vi "EOL CAN_Init CAL.vi"(7 "Flash Size":i32, 8 "Glass?":bool=TRUE, 9 "Read Session in":refnum<k21>, 10 "DSC Write Session in":refnum<k21>, 11 "SA2 Operator":T1[](array[typedef]) {"Wert" format="%.0x"}) -> (1 "Error String Out":string, 2 "TxRx Data":string[][](array[string]), 3 "Response Good?":bool)   [LabVIEW 2014]
uses:
  Typedefs/Diagnose_SA2_Rechnenbefehl.ctl
  Typedefs/Diagnose_SA2_Operation_ENUM.ctl
  Typedefs/Select Session.ctl
  <vilib>/xnet/xnet.llb/XNET Frame CAN.ctl
  <vilib>/xnet/xnet.llb/XNET Frame Type CAN.ctl
panel:
  in  "Error String":string
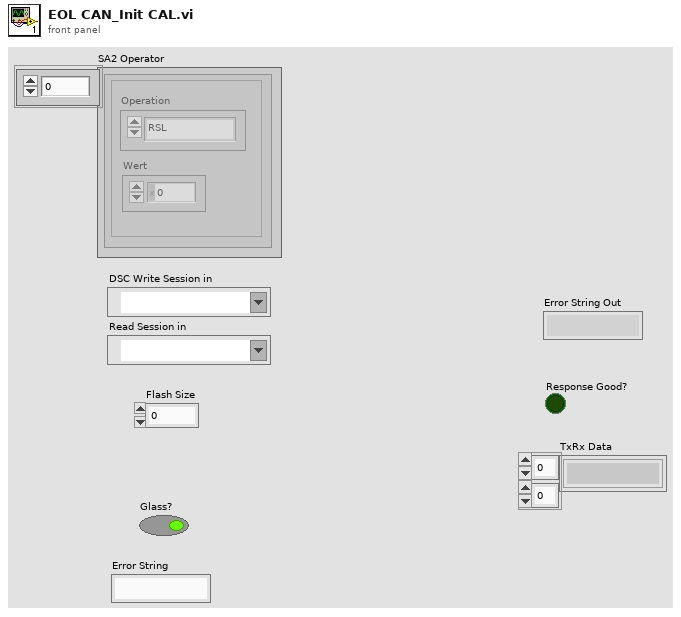
[diagram p1: front panel]
types:
  T1 = typedef "Diagnose_SA2_Rechnenbefehl.ctl" = cluster{"Operation":T2, "Wert":u32}
  T2 = typedef "Diagnose_SA2_Operation_ENUM.ctl" = enum16{"RSL", "RSR", "ADD", "SUB", "EOR", "Durchläufe", "NEXT", "BCC", "BRA", "Fertig"}
  T3 = cluster{"DSC Write Session in":refnum<k21>, "Read Session in":refnum<k21>, "Error String":string, "Response Good?":bool, "Glass?":bool, "TxRx Data":string[][], "SA2 Operator":T1[], "Flash Size":i32}
  T4 = typedef "Select Session.ctl" = enum16{"DefaultSession", "Development", "Extended", "EOL", "Programming"}
  T5 = typedef "XNET Frame CAN.ctl" = cluster{"timestamp":timestamp, "payload":u8[], "identifier":u32, "type":T6, "extended?":bool, "echo?":bool}
  T6 = typedef "XNET Frame Type CAN.ctl" = u8
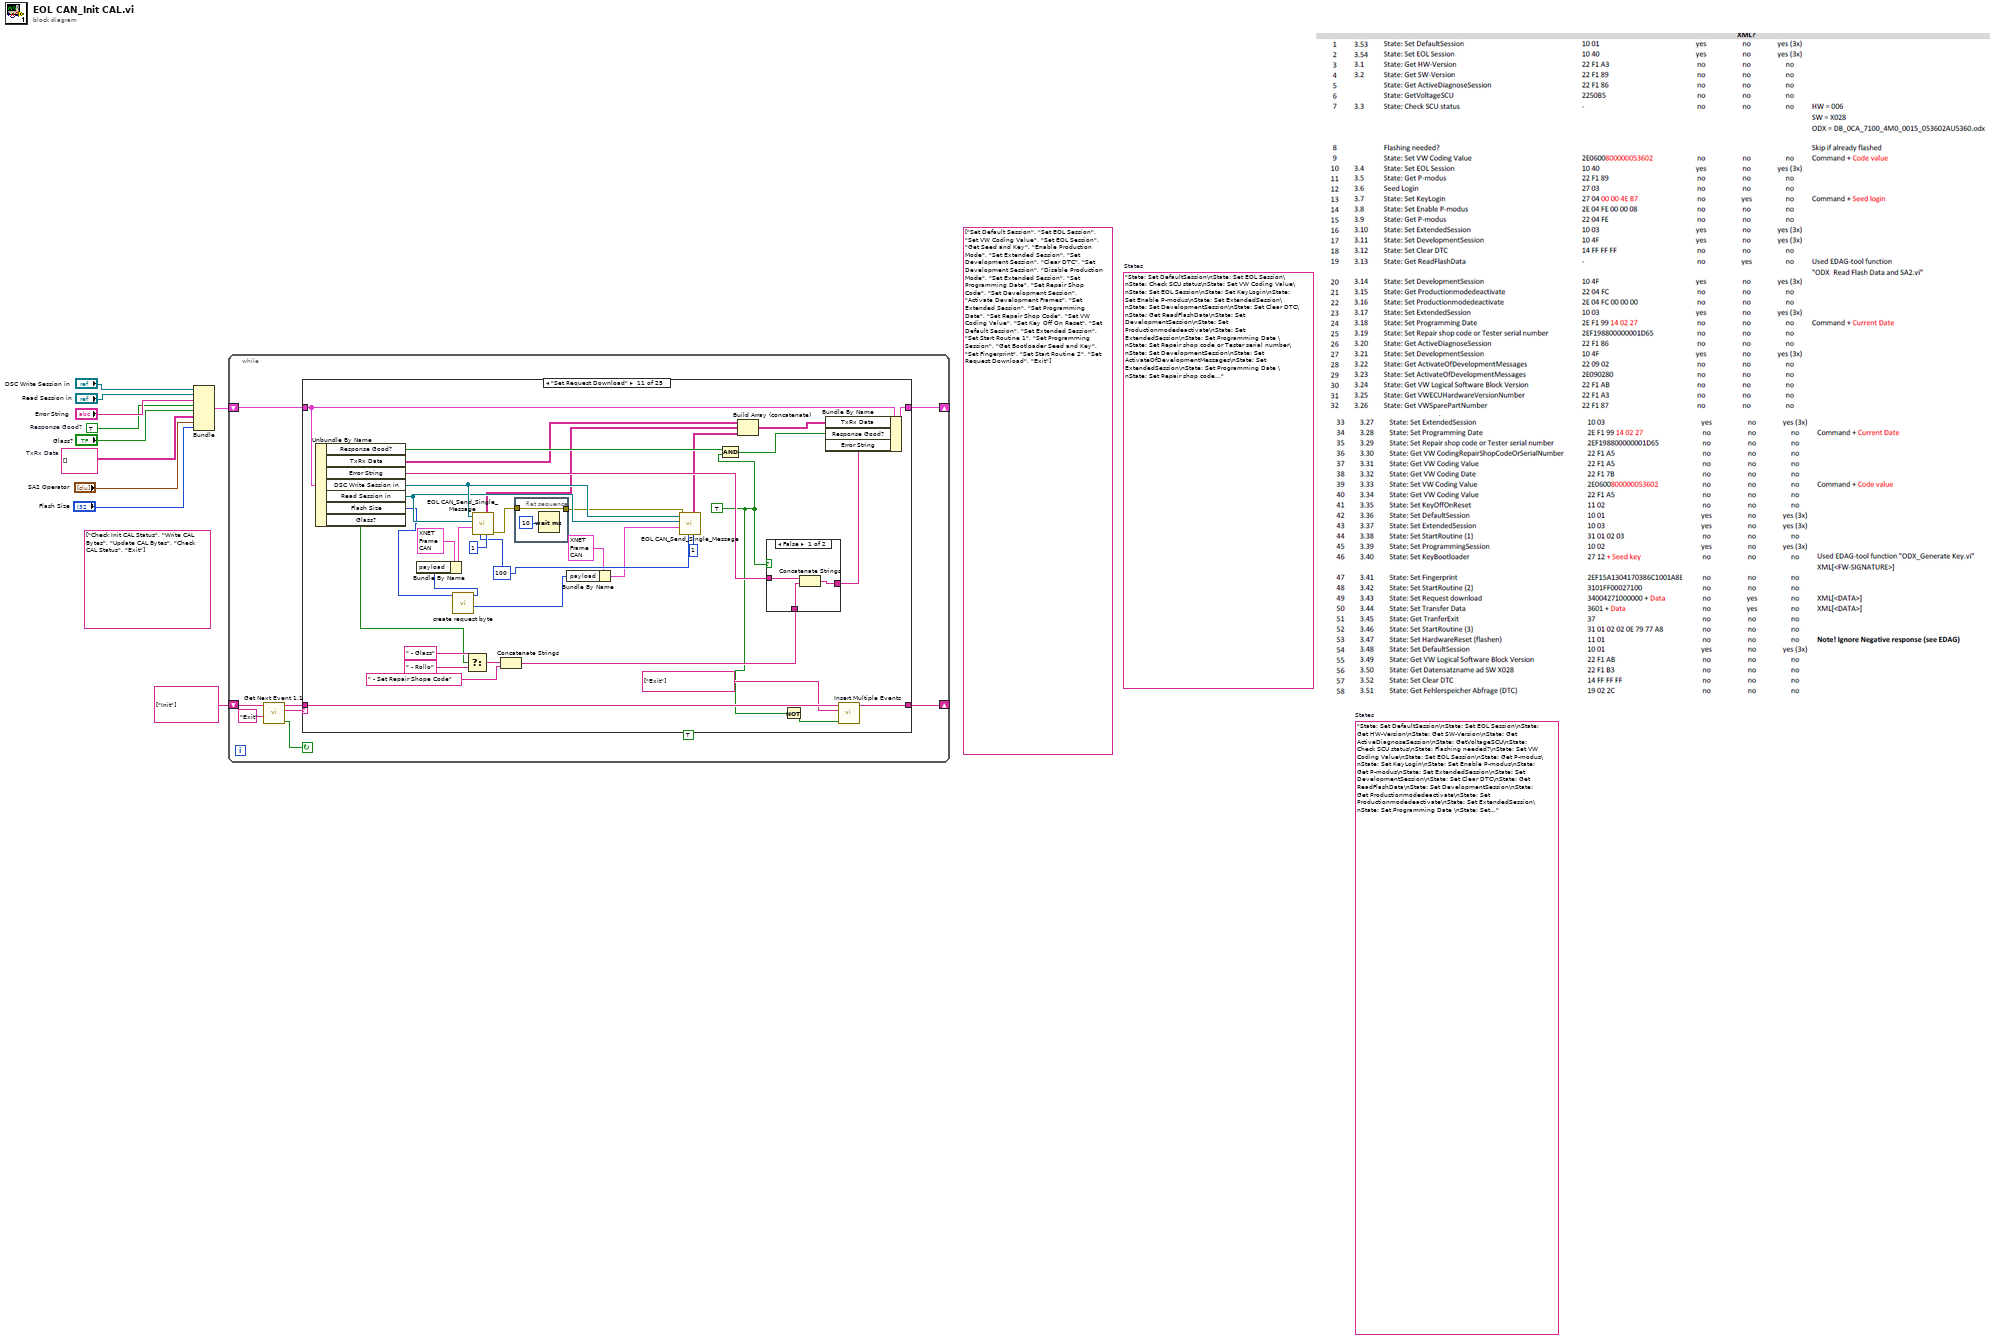
[diagram p0: block diagram]
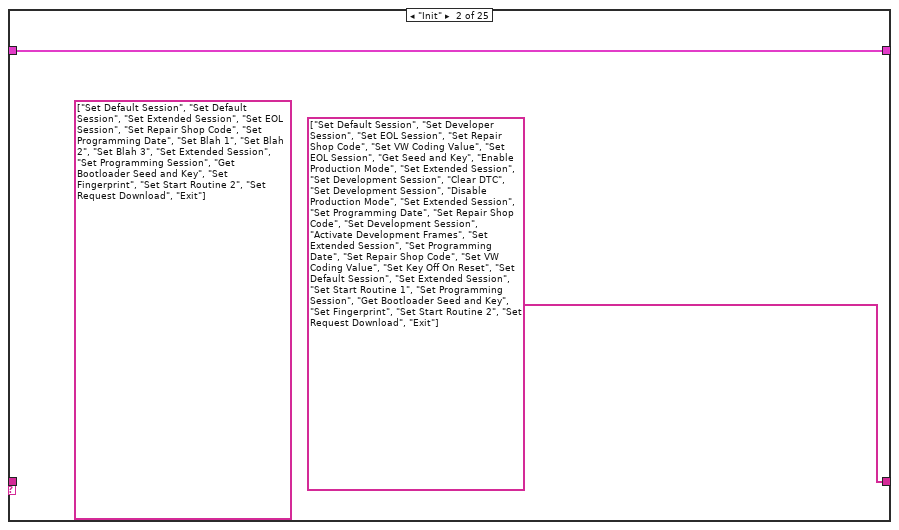
[diagram p3: hidden frame]
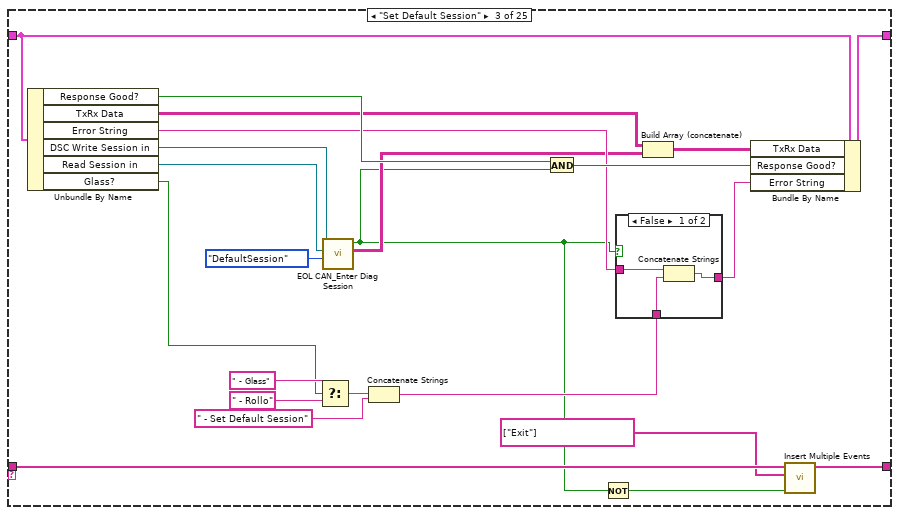
[diagram p4: hidden frame]
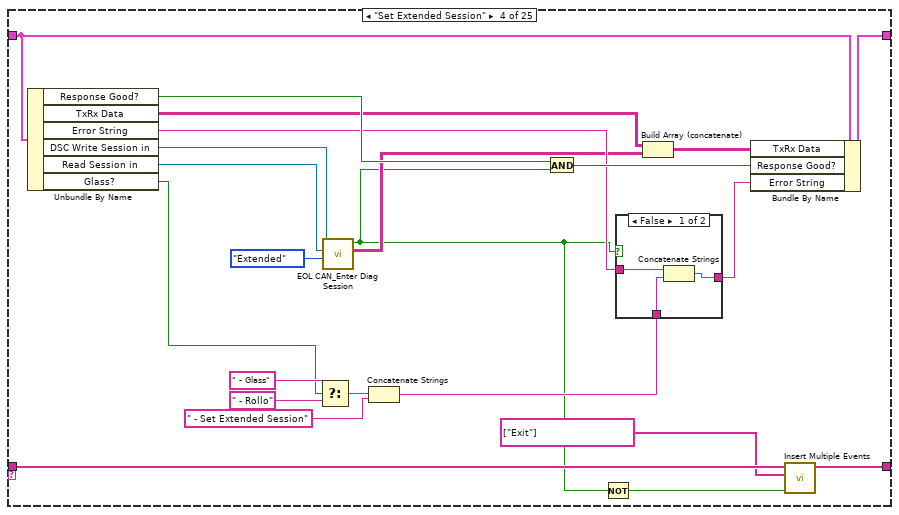
[diagram p6: hidden frame]
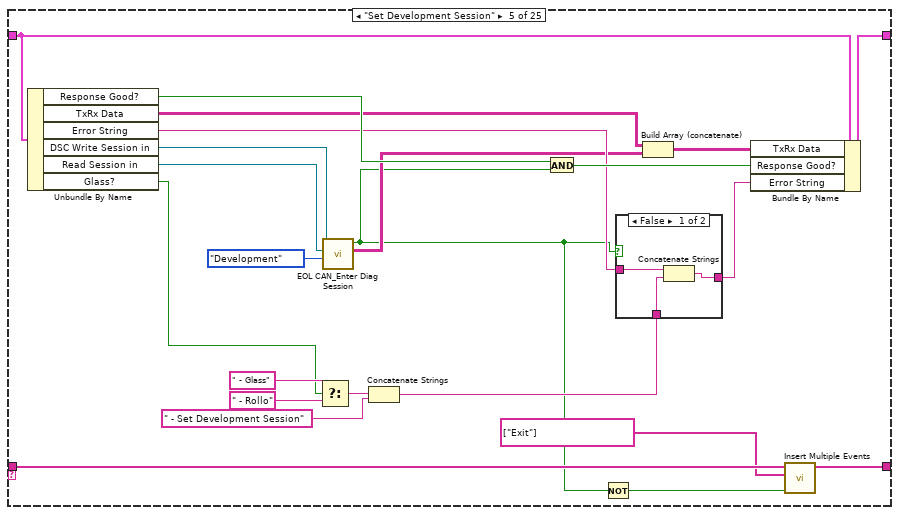
[diagram p8: hidden frame]
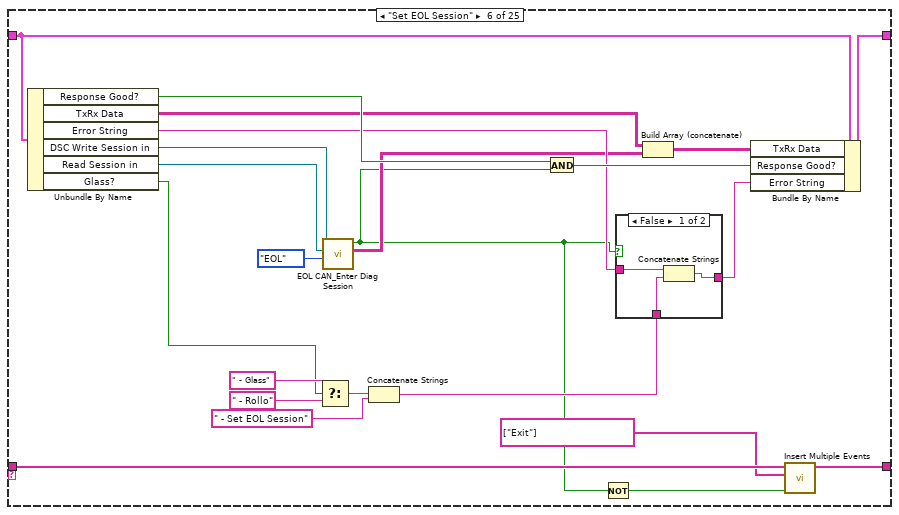
[diagram p10: hidden frame]
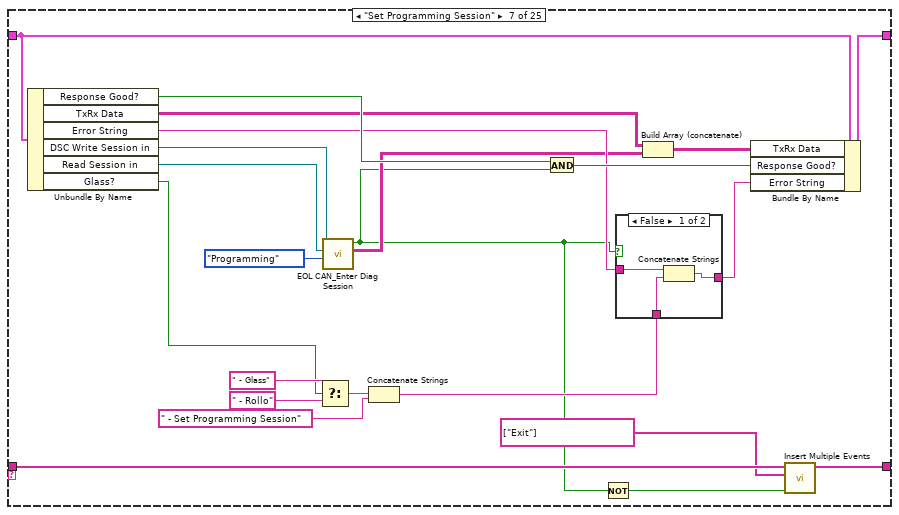
[diagram p12: hidden frame]
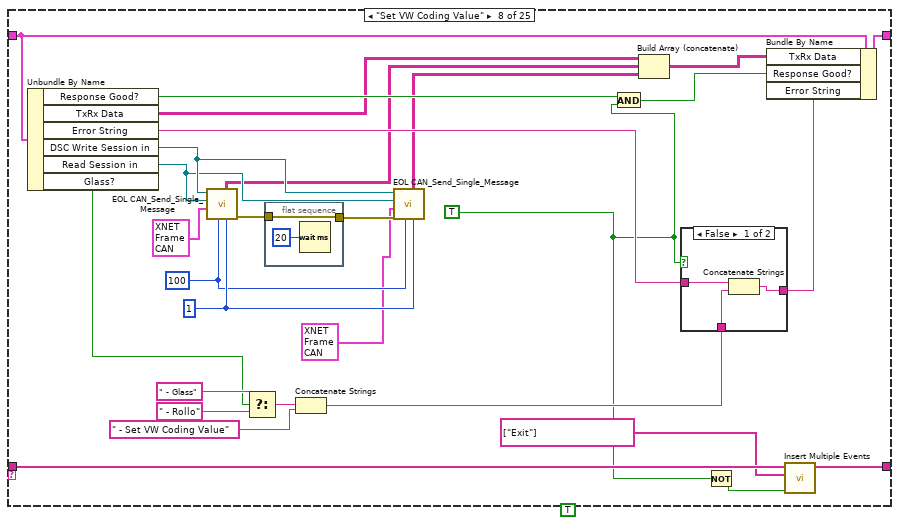
[diagram p14: hidden frame]
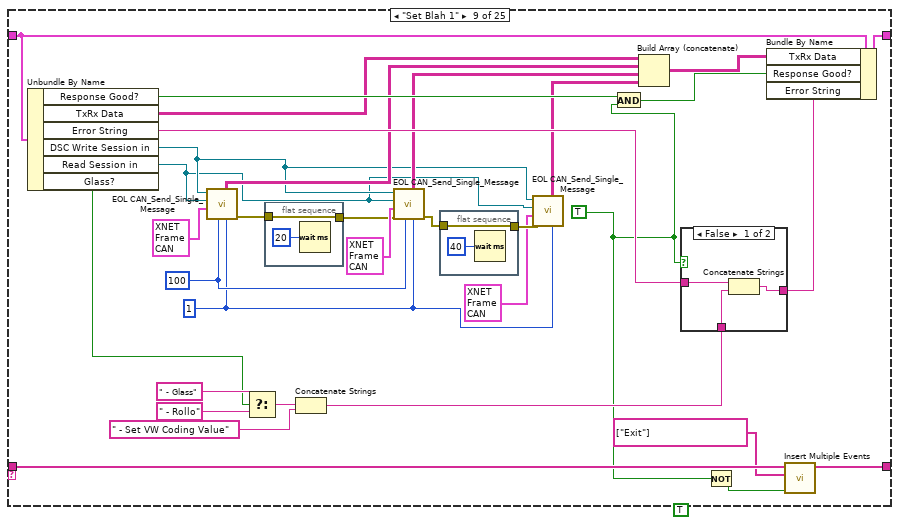
[diagram p16: hidden frame]
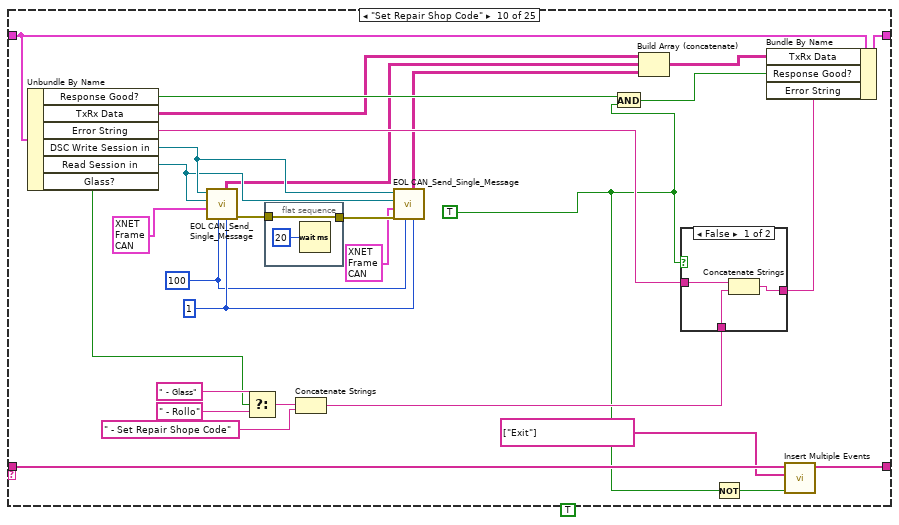
[diagram p18: hidden frame]
diagram:
  (unwired) "State: Set DefaultSession\nState: Set EOL Session\nState: Get HW-Version\nState: Get SW-Version\nState: Get ActiveDiagnoseSession\nState: GetVoltageSCU\nState: Check SCU status\nState: Flashing needed?\nState: Set VW Coding Value\nState: Set EOL Session\nState: Get P-modus\nState: Set KeyLogin\nState: Set Enable P-modus\nState: Get P-modus\nState: Set ExtendedSession\nState: Set DevelopmentSession\nState: Set Clear DTC\nState: Get ReadFlashData\nState: Set DevelopmentSession\nState: Get Productionmodedeactivate\nState: Set Productionmodedeactivate\nState: Set ExtendedSession\nState: Set Programming Date \nState: Set Repair shop code or Tester serial number\nState: Get ActiveDiagnoseSession \nState: Set DevelopmentSession\nState: Get ActivateOfDevelopmentMessages\nState: Set ActivateOfDevelopmentMessages\nState: Get VW Logical Software Block Version\nState: Get VWECUHardwareVersionNumber\nState: Get VWSparePartNumber\nState: Set ExtendedSession\nState: Set Programming Date \nState: Set Repair shop code or Tester serial number\nState: Get VW CodingRepairShopCodeOrSerialNumber\nState: Get VW Coding Value\nState: Get VW Coding Date\nState: Set VW Coding Value\nState: Get VW Coding Value\nState: Set KeyOffOnReset\nState: Set DefaultSession\nState: Set ExtendedSession\nState: Set StartRoutine (1)\nState: Set ProgrammingSession\nState: Set KeyBootloader\nState: Set Fingerprint\nState: Set StartRoutine (2)\nState: Set Request download\nState: Set Transfer Data\nState: Get TranferExit\nState: Set StartRoutine (3)\nState: Get ActiveDiagnoseSession \nState: Set HardwareReset (flashen)\nState: Set DefaultSession\nState: Get VW Logical Software Block Version\nState: Get Datensatzname ad SW X028\nState: Set Clear DTC\nState: Get DTC (TestFailed + Confirmed DTC)\nExit"  # States
  (unwired) "State: Set DefaultSession\nState: Set EOL Session\nState: Check SCU status\nState: Set VW Coding Value\nState: Set EOL Session\nState: Set KeyLogin\nState: Set Enable P-modus\nState: Set ExtendedSession\nState: Set DevelopmentSession\nState: Set Clear DTC\nState: Get ReadFlashData\nState: Set DevelopmentSession\nState: Set Productionmodedeactivate\nState: Set ExtendedSession\nState: Set Programming Date \nState: Set Repair shop code or Tester serial number\nState: Set DevelopmentSession\nState: Set ActivateOfDevelopmentMessages\nState: Set ExtendedSession\nState: Set Programming Date \nState: Set Repair shop code or Tester serial number\nState: Set VW Coding Value\nState: Set KeyOffOnReset\nState: Set DefaultSession\nState: Set ExtendedSession\nState: Set StartRoutine (1)\nState: Set ProgrammingSession\nState: Set KeyBootloader\nState: Set Fingerprint\nState: Set StartRoutine (2)\nState: Set Request download\nState: Set Transfer Data\nState: Get TranferExit\nState: Set StartRoutine (3)\nState: Set HardwareReset (flashen)\nState: Set DefaultSession\nState: Get Datensatzname ad SW X028\nState: Set Clear DTC\nState: Get DTC (TestFailed + Confirmed DTC)\nExit"  # States
  (unwired) string[] ["Set Default Session", "Set EOL Session", "Set VW Coding Value", "Set EOL Session", "Get Seed and Key", "Enable Production Mode", "Set Extended Session", "Set Development Session", "Clear DTC", "Set Development Session", "Disable Production Mode", "Set Extended Session", "Set Programming Date", "Set Repair Shop Code", "Set Development Session", "Activate Development Frames", "Set Extended Session", "Set Programming Date", "Set Repair Shop Code", "Set VW Coding Value", "Set Key Off On Reset", "Set Default Session", "Set Extended Session", "Set Start Routine 1", "Set Programming Session", "Get Bootloader Seed and Key", "Set Fingerprint", "Set Start Routine 2", "Set Request Download", "Exit"] ("event queue out")
  (unwired) string[] ["Check Init CAL Status", "Write CAL Bytes", "Update CAL Bytes", "Check CAL Status", "Exit"] ("event queue out")
  w5 = string[][] []  # TxRx Data
  w8 = TRUE  # Response Good?
  n1 = Bundle("DSC Write Session in"="DSC Write Session in", "Read Session in"="Read Session in", "Error String"="Error String", "Response Good?"=w8, "Glass?"="Glass?", "TxRx Data"=w5, "SA2 Operator"="SA2 Operator", "Flash Size"="Flash Size") -> (w7:T3)  [unwired: 1 in]
  n2 = while {
    shift-right: [w16] -> _
    shift-left: string[] ["Init"] ("event queue out") -> [w15]
    shift-right: [w13] -> _
    shift-left: w7 -> [w14]
    stop <- w18 continue-if-true
    n3 = call "Get Next Event 1.1.vi"("Exit Event"="Exit", "event queue in"=w15) -> ("Condition (Exit:F)"=w18:bool, "next event"=w11:string, "event queue out"=w17:string[])  [unwired: 6 in, 1 out]
    n4 = case shown="\"Set Request Download\"" w11 {
      tunnel: w17 -> [w20 _ w33 w60 w87 w114 w141 w174 w213 w250 w291 w326 w354 w381 w407 w433 w470 w500 w531 w560 w587 w614 w641 w667 w688]
      tunnel: [w20 string[] ["Set Default Session", "Set Developer Session", "Set EOL Session", "Set Repair Shop Code", "Set VW Coding Value", "Set EOL Session", "Get Seed and Key", "Enable Production Mode", "Set Extended Session", "Set Development Session", "Clear DTC", "Set Development Session", "Disable Production Mode", "Set Extended Session", "Set Programming Date", "Set Repair Shop Code", "Set Development Session", "Activate Development Frames", "Set Extended Session", "Set Programming Date", "Set Repair Shop Code", "Set VW Coding Value", "Set Key Off On Reset", "Set Default Session", "Set Extended Session", "Set Start Routine 1", "Set Programming Session", "Get Bootloader Seed and Key", "Set Fingerprint", "Set Start Routine 2", "Set Request Download", "Exit"] ("event queue out") w34 w61 w88 w115 w142 w175 w214 w251 w292 w327 w355 w382 w408 w434 w471 w501 w532 w561 w588 w615 w642 w668 w688] -> w16
      tunnel: w14 -> [w19 w22 w44 w71 w98 w125 w152 w185 w224 w261 w302 w337 w365 w392 w418 w444 w481 w511 w542 w571 w598 w625 w652 w678 w687]
      tunnel: [w19 w22 w42 w69 w96 w123 w150 w183 w222 w259 w300 w335 w363 w390 w416 w442 w479 w509 w540 w569 w596 w623 w650 w676 w687] -> w13
      frame "Error", Default {
      }
      frame "Init" {
        (unwired) string[] ["Set Default Session", "Set Default Session", "Set Extended Session", "Set EOL Session", "Set Repair Shop Code", "Set Programming Date", "Set Blah 1", "Set Blah 2", "Set Blah 3", "Set Extended Session", "Set Programming Session", "Get Bootloader Seed and Key", "Set Fingerprint", "Set Start Routine 2", "Set Request Download", "Exit"] ("event queue out")
        # "Inalfa Sequences"
        # "Conti-Sequences"
      }
      frame "Set Default Session" {
        n5 = Unbundle By Name(w44) -> ("Response Good?"=w45:bool, "TxRx Data"=w31:string[][], "Error String"=w41:string, "DSC Write Session in"=w28:refnum<k21>, "Read Session in"=w27:refnum<k21>, "Glass?"=w25:bool)
        n6 = Select(t=" - Glass" ("Error Description"), s=w25, f=" - Rollo" ("Error Description")) -> (s? t:f=w39:string)
        n7 = call "EOL CAN_Enter Diag Session.vi"("Session"=Select_Session."DefaultSession", "Read Session in"=w27, "Write Session in"=w28) -> ("TxRx Data"=w29:string[][], "Response Good?"=w24:bool)  [unwired: 6 in, 1 out]
        n8 = Concatenate Strings(w39, " - Set Default Session" ("Error Description")) -> (w35:string)
        n9 = And(x=w45, y=w24) -> (x .and. y?=w43:bool)
        n10 = Not(x=w24) -> (.not. x?=w23:bool)
        n11 = case shown="False" w24 {
          tunnel: w41 -> [w47 w49]
          tunnel: [w48 w49] -> w40
          tunnel: w35 -> [w46 _]
          frame False {
            n12 = Concatenate Strings(w47, w46) -> (w48:string)
          }
          frame True {
          }
        }
        n13 = Build Array (concatenate)(w31, w29) -> (w30:string[][])
        n14 = Bundle By Name(cluster=w44, "TxRx Data"=w30, "Response Good?"=w43, "Error String"=w40) -> (w42:T3)
        n15 = call "Insert Multiple Events.vi"("Insert all? (T)"=w23, "Events to Insert"=string[] ["Exit"], "Event queue in"=w33) -> ("Event queue out"=w34:string[])  [unwired: 4 in]
      }
      frame "Set Extended Session" {
        n16 = Unbundle By Name(w71) -> ("Response Good?"=w72:bool, "TxRx Data"=w58:string[][], "Error String"=w68:string, "DSC Write Session in"=w55:refnum<k21>, "Read Session in"=w54:refnum<k21>, "Glass?"=w52:bool)
        n17 = Select(t=" - Glass" ("Error Description"), s=w52, f=" - Rollo" ("Error Description")) -> (s? t:f=w66:string)
        n18 = call "EOL CAN_Enter Diag Session.vi"("Session"=Select_Session."Extended", "Read Session in"=w54, "Write Session in"=w55) -> ("TxRx Data"=w56:string[][], "Response Good?"=w51:bool)  [unwired: 6 in, 1 out]
        n19 = Concatenate Strings(w66, " - Set Extended Session" ("Error Description")) -> (w62:string)
        n20 = And(x=w72, y=w51) -> (x .and. y?=w70:bool)
        n21 = Not(x=w51) -> (.not. x?=w50:bool)
        n22 = case shown="False" w51 {
          tunnel: w68 -> [w74 w76]
          tunnel: [w75 w76] -> w67
          tunnel: w62 -> [w73 _]
          frame False {
            n23 = Concatenate Strings(w74, w73) -> (w75:string)
          }
          frame True {
          }
        }
        n24 = Build Array (concatenate)(w58, w56) -> (w57:string[][])
        n25 = Bundle By Name(cluster=w71, "TxRx Data"=w57, "Response Good?"=w70, "Error String"=w67) -> (w69:T3)
        n26 = call "Insert Multiple Events.vi"("Insert all? (T)"=w50, "Events to Insert"=string[] ["Exit"], "Event queue in"=w60) -> ("Event queue out"=w61:string[])  [unwired: 4 in]
      }
      frame "Set Development Session" {
        n27 = Unbundle By Name(w98) -> ("Response Good?"=w99:bool, "TxRx Data"=w85:string[][], "Error String"=w95:string, "DSC Write Session in"=w82:refnum<k21>, "Read Session in"=w81:refnum<k21>, "Glass?"=w79:bool)
        n28 = Select(t=" - Glass" ("Error Description"), s=w79, f=" - Rollo" ("Error Description")) -> (s? t:f=w93:string)
        n29 = call "EOL CAN_Enter Diag Session.vi"("Session"=Select_Session."Development", "Read Session in"=w81, "Write Session in"=w82) -> ("TxRx Data"=w83:string[][], "Response Good?"=w78:bool)  [unwired: 6 in, 1 out]
        n30 = Concatenate Strings(w93, " - Set Development Session" ("Error Description")) -> (w89:string)
        n31 = And(x=w99, y=w78) -> (x .and. y?=w97:bool)
        n32 = Not(x=w78) -> (.not. x?=w77:bool)
        n33 = case shown="False" w78 {
          tunnel: w95 -> [w101 w103]
          tunnel: [w102 w103] -> w94
          tunnel: w89 -> [w100 _]
          frame False {
            n34 = Concatenate Strings(w101, w100) -> (w102:string)
          }
          frame True {
          }
        }
        n35 = Build Array (concatenate)(w85, w83) -> (w84:string[][])
        n36 = Bundle By Name(cluster=w98, "TxRx Data"=w84, "Response Good?"=w97, "Error String"=w94) -> (w96:T3)
        n37 = call "Insert Multiple Events.vi"("Insert all? (T)"=w77, "Events to Insert"=string[] ["Exit"], "Event queue in"=w87) -> ("Event queue out"=w88:string[])  [unwired: 4 in]
      }
      frame "Set EOL Session" {
        n38 = Unbundle By Name(w125) -> ("Response Good?"=w126:bool, "TxRx Data"=w112:string[][], "Error String"=w122:string, "DSC Write Session in"=w109:refnum<k21>, "Read Session in"=w108:refnum<k21>, "Glass?"=w106:bool)
        n39 = Select(t=" - Glass" ("Error Description"), s=w106, f=" - Rollo" ("Error Description")) -> (s? t:f=w120:string)
        n40 = call "EOL CAN_Enter Diag Session.vi"("Session"=Select_Session."EOL", "Read Session in"=w108, "Write Session in"=w109) -> ("TxRx Data"=w110:string[][], "Response Good?"=w105:bool)  [unwired: 6 in, 1 out]
        n41 = Concatenate Strings(w120, " - Set EOL Session" ("Error Description")) -> (w116:string)
        n42 = And(x=w126, y=w105) -> (x .and. y?=w124:bool)
        n43 = Not(x=w105) -> (.not. x?=w104:bool)
        n44 = case shown="False" w105 {
          tunnel: w122 -> [w128 w130]
          tunnel: [w129 w130] -> w121
          tunnel: w116 -> [w127 _]
          frame False {
            n45 = Concatenate Strings(w128, w127) -> (w129:string)
          }
          frame True {
          }
        }
        n46 = Build Array (concatenate)(w112, w110) -> (w111:string[][])
        n47 = Bundle By Name(cluster=w125, "TxRx Data"=w111, "Response Good?"=w124, "Error String"=w121) -> (w123:T3)
        n48 = call "Insert Multiple Events.vi"("Insert all? (T)"=w104, "Events to Insert"=string[] ["Exit"], "Event queue in"=w114) -> ("Event queue out"=w115:string[])  [unwired: 4 in]
      }
      frame "Set Programming Session" {
        n49 = Unbundle By Name(w152) -> ("Response Good?"=w153:bool, "TxRx Data"=w139:string[][], "Error String"=w149:string, "DSC Write Session in"=w136:refnum<k21>, "Read Session in"=w135:refnum<k21>, "Glass?"=w133:bool)
        n50 = Select(t=" - Glass" ("Error Description"), s=w133, f=" - Rollo" ("Error Description")) -> (s? t:f=w147:string)
        n51 = call "EOL CAN_Enter Diag Session.vi"("Session"=Select_Session."Programming", "Read Session in"=w135, "Write Session in"=w136) -> ("TxRx Data"=w137:string[][], "Response Good?"=w132:bool)  [unwired: 6 in, 1 out]
        n52 = Concatenate Strings(w147, " - Set Programming Session" ("Error Description")) -> (w143:string)
        n53 = And(x=w153, y=w132) -> (x .and. y?=w151:bool)
        n54 = Not(x=w132) -> (.not. x?=w131:bool)
        n55 = case shown="False" w132 {
          tunnel: w149 -> [w155 w157]
          tunnel: [w156 w157] -> w148
          tunnel: w143 -> [w154 _]
          frame False {
            n56 = Concatenate Strings(w155, w154) -> (w156:string)
          }
          frame True {
          }
        }
        n57 = Build Array (concatenate)(w139, w137) -> (w138:string[][])
        n58 = Bundle By Name(cluster=w152, "TxRx Data"=w138, "Response Good?"=w151, "Error String"=w148) -> (w150:T3)
        n59 = call "Insert Multiple Events.vi"("Insert all? (T)"=w131, "Events to Insert"=string[] ["Exit"], "Event queue in"=w141) -> ("Event queue out"=w142:string[])  [unwired: 4 in]
      }
      frame "Set VW Coding Value" {
        w159 = TRUE ("Response Good?")
        (unwired) TRUE ("Insert all? (T)")
        w166 = 1 ("Retries")
        w165 = u32 100 ("Msg Wait Time")
        n60 = Unbundle By Name(w185) -> ("Response Good?"=w186:bool, "TxRx Data"=w172:string[][], "Error String"=w182:string, "DSC Write Session in"=w168:refnum<k21>, "Read Session in"=w167:refnum<k21>, "Glass?"=w170:bool)
        n61 = call "EOL CAN_Send_Single_Message.vi"("Retries"=w166, "Msg Wait Time"=w165, "Tx CAN frame"=T5 {"timestamp"=timestamp(0 s since 1904-01-01), "payload"=[16, 9, 46, 6, 0, 2, 0, 0], "identifier"=402391172, "type"=8, "extended?"=TRUE, "echo?"=FALSE}, "Read Session in"=w167, "Write Session in"=w168) -> ("Error out"=w162:errorcluster, "TxRx Data"=w164:string[][])  [unwired: 2 in, 3 out]
        n62 = Select(t=" - Glass" ("Error Description"), s=w170, f=" - Rollo" ("Error Description")) -> (s? t:f=w180:string)
        n63 = flat-sequence {
          tunnel: w162 -> [w188]
          tunnel: [w188] -> w161
          frame #0 {
            n64 = Wait (ms)(milliseconds to wait=u32 20) -> ()  [unwired: 1 out]
          }
        }
        n65 = Concatenate Strings(w180, " - Set VW Coding Value" ("Error Description")) -> (w176:string)
        n66 = call "EOL CAN_Send_Single_Message.vi"("Retries"=w166, "Msg Wait Time"=w165, "Error in"=w161, "Tx CAN frame"=T5 {"timestamp"=timestamp(0 s since 1904-01-01), "payload"=[33, 115, 113, 11, 85, 85, 85, 85], "identifier"=402391172, "type"=8, "extended?"=TRUE, "echo?"=FALSE}, "Read Session in"=w167, "Write Session in"=w168) -> ("TxRx Data"=w163:string[][])  [unwired: 1 in, 4 out]
        n67 = And(x=w186, y=w159) -> (x .and. y?=w184:bool)
        n68 = Build Array (concatenate)(w172, w164, w163) -> (w171:string[][])
        n69 = case shown="False" w159 {
          tunnel: w182 -> [w190 w192]
          tunnel: [w191 w192] -> w181
          tunnel: w176 -> [w189 _]
          frame False {
            n70 = Concatenate Strings(w190, w189) -> (w191:string)
          }
          frame True {
          }
        }
        n71 = Not(x=w159) -> (.not. x?=w160:bool)
        n72 = Bundle By Name(cluster=w185, "TxRx Data"=w171, "Response Good?"=w184, "Error String"=w181) -> (w183:T3)
        n73 = call "Insert Multiple Events.vi"("Insert all? (T)"=w160, "Events to Insert"=string[] ["Exit"], "Event queue in"=w174) -> ("Event queue out"=w175:string[])  [unwired: 4 in]
      }
      frame "Set Blah 1" {
        w200 = TRUE ("Response Good?")
        (unwired) TRUE ("Insert all? (T)")
        w193 = 1 ("Retries")
        w206 = u32 100 ("Msg Wait Time")
        n74 = Unbundle By Name(w224) -> ("Response Good?"=w225:bool, "TxRx Data"=w211:string[][], "Error String"=w221:string, "DSC Write Session in"=w197:refnum<k21>, "Read Session in"=w196:refnum<k21>, "Glass?"=w209:bool)
        n75 = call "EOL CAN_Send_Single_Message.vi"("Retries"=w193, "Msg Wait Time"=w206, "Tx CAN frame"=T5 {"timestamp"=timestamp(0 s since 1904-01-01), "payload"=[16, 14, 46, 241, 160, 67, 111, 110], "identifier"=402391172, "type"=8, "extended?"=TRUE, "echo?"=FALSE}, "Read Session in"=w196, "Write Session in"=w197) -> ("Error out"=w203:errorcluster, "TxRx Data"=w205:string[][])  [unwired: 2 in, 3 out]
        n76 = Select(t=" - Glass" ("Error Description"), s=w209, f=" - Rollo" ("Error Description")) -> (s? t:f=w219:string)
        n77 = flat-sequence {
          tunnel: w203 -> [w229]
          tunnel: [w229] -> w202
          frame #0 {
            n78 = Wait (ms)(milliseconds to wait=u32 20) -> ()  [unwired: 1 out]
          }
        }
        n79 = Concatenate Strings(w219, " - Set VW Coding Value" ("Error Description")) -> (w215:string)
        n80 = call "EOL CAN_Send_Single_Message.vi"("Retries"=w193, "Msg Wait Time"=w206, "Error in"=w202, "Tx CAN frame"=T5 {"timestamp"=timestamp(0 s since 1904-01-01), "payload"=[33, 116, 105, 110, 101, 110, 116, 97], "identifier"=402391172, "type"=8, "extended?"=TRUE, "echo?"=FALSE}, "Read Session in"=w196, "Write Session in"=w197) -> ("Error out"=w199:errorcluster, "TxRx Data"=w204:string[][])  [unwired: 1 in, 3 out]
        n81 = flat-sequence {
          tunnel: w199 -> [w227]
          tunnel: [w227] -> w198
          frame #0 {
            n82 = Wait (ms)(milliseconds to wait=u32 40) -> ()  [unwired: 1 out]
          }
        }
        n83 = call "EOL CAN_Send_Single_Message.vi"("Retries"=w193, "Error in"=w198, "Tx CAN frame"=T5 {"timestamp"=timestamp(0 s since 1904-01-01), "payload"=[34, 108, 85, 85, 85, 85, 85, 85], "identifier"=402391172, "type"=8, "extended?"=TRUE, "echo?"=FALSE}, "Read Session in"=w196, "Write Session in"=w197) -> ("TxRx Data"=w194:string[][])  [unwired: 2 in, 4 out]
        n84 = And(x=w225, y=w200) -> (x .and. y?=w223:bool)
        n85 = Build Array (concatenate)(w211, w205, w204, w194) -> (w210:string[][])
        n86 = case shown="False" w200 {
          tunnel: w221 -> [w231 w233]
          tunnel: [w232 w233] -> w220
          tunnel: w215 -> [w230 _]
          frame False {
            n87 = Concatenate Strings(w231, w230) -> (w232:string)
          }
          frame True {
          }
        }
        n88 = Not(x=w200) -> (.not. x?=w201:bool)
        n89 = Bundle By Name(cluster=w224, "TxRx Data"=w210, "Response Good?"=w223, "Error String"=w220) -> (w222:T3)
        n90 = call "Insert Multiple Events.vi"("Insert all? (T)"=w201, "Events to Insert"=string[] ["Exit"], "Event queue in"=w213) -> ("Event queue out"=w214:string[])  [unwired: 4 in]
      }
      frame "Set Repair Shop Code" {
        w236 = TRUE ("Response Good?")
        (unwired) TRUE ("Insert all? (T)")
        w243 = 1 ("Retries")
        w242 = u32 100 ("Msg Wait Time")
        n91 = Unbundle By Name(w261) -> ("Response Good?"=w262:bool, "TxRx Data"=w248:string[][], "Error String"=w258:string, "DSC Write Session in"=w245:refnum<k21>, "Read Session in"=w244:refnum<k21>, "Glass?"=w246:bool)
        n92 = call "EOL CAN_Send_Single_Message.vi"("Retries"=w243, "Msg Wait Time"=w242, "Tx CAN frame"=T5 {"timestamp"=timestamp(0 s since 1904-01-01), "payload"=[16, 9, 46, 241, 152, 128, 0, 0], "identifier"=402391172, "type"=8, "extended?"=TRUE, "echo?"=FALSE}, "Read Session in"=w244, "Write Session in"=w245) -> ("Error out"=w239:errorcluster, "TxRx Data"=w241:string[][])  [unwired: 2 in, 3 out]
        n93 = Select(t=" - Glass" ("Error Description"), s=w246, f=" - Rollo" ("Error Description")) -> (s? t:f=w256:string)
        n94 = flat-sequence {
          tunnel: w239 -> [w264]
          tunnel: [w264] -> w238
          frame #0 {
            n95 = Wait (ms)(milliseconds to wait=u32 20) -> ()  [unwired: 1 out]
          }
        }
        n96 = Concatenate Strings(w256, " - Set Repair Shope Code" ("Error Description")) -> (w252:string)
        n97 = call "EOL CAN_Send_Single_Message.vi"("Retries"=w243, "Msg Wait Time"=w242, "Error in"=w238, "Tx CAN frame"=T5 {"timestamp"=timestamp(0 s since 1904-01-01), "payload"=[33, 0, 29, 101, 85, 85, 85, 85], "identifier"=402391172, "type"=8, "extended?"=TRUE, "echo?"=FALSE}, "Read Session in"=w244, "Write Session in"=w245) -> ("TxRx Data"=w240:string[][])  [unwired: 1 in, 4 out]
        n98 = And(x=w262, y=w236) -> (x .and. y?=w260:bool)
        n99 = Build Array (concatenate)(w248, w241, w240) -> (w247:string[][])
        n100 = case shown="False" w236 {
          tunnel: w258 -> [w266 w268]
          tunnel: [w267 w268] -> w257
          tunnel: w252 -> [w265 _]
          frame False {
            n101 = Concatenate Strings(w266, w265) -> (w267:string)
          }
          frame True {
          }
        }
        n102 = Not(x=w236) -> (.not. x?=w237:bool)
        n103 = Bundle By Name(cluster=w261, "TxRx Data"=w247, "Response Good?"=w260, "Error String"=w257) -> (w259:T3)
        n104 = call "Insert Multiple Events.vi"("Insert all? (T)"=w237, "Events to Insert"=string[] ["Exit"], "Event queue in"=w250) -> ("Event queue out"=w251:string[])  [unwired: 4 in]
      }
      frame "Set Request Download" {
        w277 = TRUE
        (unwired) TRUE ("Insert all? (T)")
        w283 = u32 100 ("Msg Wait Time")
        n105 = Unbundle By Name(w302) -> ("Response Good?"=w303:bool, "TxRx Data"=w289:string[][], "Error String"=w299:string, "DSC Write Session in"=w286:refnum<k21>, "Read Session in"=w285:refnum<k21>, "Flash Size"=w274:i32, "Glass?"=w287:bool)
        n106 = call "create request byte.vi"("x"=w274) -> ("output array 2"=w270:u8[], "output array"=w273:u8[])  [unwired: 9 in]
        n107 = Bundle By Name(cluster=T5 {"timestamp"=timestamp(0 s since 1904-01-01), "payload"=[16, 9, 52, 0, 66, 0, 0, 0], "identifier"=402391172, "type"=8, "extended?"=TRUE, "echo?"=FALSE} ("Tx CAN frame"), "payload"=w273) -> (w275:T5)
        n108 = Select(t=" - Glass" ("Error Description"), s=w287, f=" - Rollo" ("Error Description")) -> (s? t:f=w297:string)
        n109 = call "EOL CAN_Send_Single_Message.vi"("Retries"=1, "Msg Wait Time"=w283, "Tx CAN frame"=w275, "Read Session in"=w285, "Write Session in"=w286) -> ("Error out"=w280:errorcluster, "TxRx Data"=w282:string[][])  [unwired: 2 in, 3 out]
        n110 = Concatenate Strings(w297, " - Set Repair Shope Code" ("Error Description")) -> (w293:string)
        n111 = flat-sequence {
          tunnel: w280 -> [w305]
          tunnel: [w305] -> w279
          frame #0 {
            n112 = Wait (ms)(milliseconds to wait=u32 10) -> ()  [unwired: 1 out]
          }
        }
        n113 = Bundle By Name(cluster=T5 {"timestamp"=timestamp(0 s since 1904-01-01), "payload"=[33, 0, 0, 0, 0, 85, 85, 85], "identifier"=402391172, "type"=8, "extended?"=TRUE, "echo?"=FALSE} ("Tx CAN frame"), "payload"=w270) -> (w271:T5)
        n114 = call "EOL CAN_Send_Single_Message.vi"("Retries"=1, "Msg Wait Time"=w283, "Error in"=w279, "Tx CAN frame"=w271, "Read Session in"=w285, "Write Session in"=w286) -> ("TxRx Data"=w281:string[][])  [unwired: 1 in, 4 out]
        n115 = And(x=w303, y=w277) -> (x .and. y?=w301:bool)
        n116 = Build Array (concatenate)(w289, w282, w281) -> (w288:string[][])
        n117 = case shown="False" w277 {
          tunnel: w299 -> [w307 w309]
          tunnel: [w308 w309] -> w298
          tunnel: w293 -> [w306 _]
          frame False {
            n118 = Concatenate Strings(w307, w306) -> (w308:string)
          }
          frame True {
          }
        }
        n119 = Not(x=w277) -> (.not. x?=w278:bool)
        n120 = Bundle By Name(cluster=w302, "TxRx Data"=w288, "Response Good?"=w301, "Error String"=w298) -> (w300:T3)
        n121 = call "Insert Multiple Events.vi"("Insert all? (T)"=w278, "Events to Insert"=string[] ["Exit"], "Event queue in"=w291) -> ("Event queue out"=w292:string[])  [unwired: 4 in]
      }
      frame "Set Fingerprint" {
        (unwired) T5 {"timestamp"=timestamp(0 s since 1904-01-01), "payload"=[16, 12, 46, 241, 90, 23, 4, 39], "identifier"=402391172, "type"=8, "extended?"=TRUE, "echo?"=FALSE} ("Tx CAN frame")
        (unwired) T5 {"timestamp"=timestamp(0 s since 1904-01-01), "payload"=[33, 60, 85, 68, 98, 103, 62, 85], "identifier"=402391172, "type"=8, "extended?"=TRUE, "echo?"=FALSE} ("Tx CAN frame")
        w311 = TRUE
        (unwired) TRUE ("Insert all? (T)")
        w319 = 1 ("Retries")
        w318 = u32 100 ("Msg Wait Time")
        n122 = Unbundle By Name(w337) -> ("Response Good?"=w338:bool, "TxRx Data"=w324:string[][], "Error String"=w334:string, "DSC Write Session in"=w321:refnum<k21>, "Read Session in"=w320:refnum<k21>, "Glass?"=w322:bool)
        n123 = Select(t=" - Glass" ("Error Description"), s=w322, f=" - Rollo" ("Error Description")) -> (s? t:f=w332:string)
        n124 = call "EOL CAN_Send_Single_Message.vi"("Retries"=w319, "Msg Wait Time"=w318, "Tx CAN frame"=T5 {"timestamp"=timestamp(0 s since 1904-01-01), "payload"=[16, 12, 46, 241, 90, 19, 4, 23], "identifier"=402391172, "type"=8, "extended?"=TRUE, "echo?"=FALSE}, "Read Session in"=w320, "Write Session in"=w321) -> ("Error out"=w315:errorcluster, "TxRx Data"=w317:string[][])  [unwired: 2 in, 3 out]
        n125 = Concatenate Strings(w332, " - Set Fingerprint" ("Error Description")) -> (w328:string)
        n126 = flat-sequence {
          tunnel: w315 -> [w340]
          tunnel: [w340] -> w314
          frame #0 {
            n127 = Wait (ms)(milliseconds to wait=u32 20) -> ()  [unwired: 1 out]
          }
        }
        n128 = call "EOL CAN_Send_Single_Message.vi"("Retries"=w319, "Msg Wait Time"=w318, "Error in"=w314, "Tx CAN frame"=T5 {"timestamp"=timestamp(0 s since 1904-01-01), "payload"=[33, 3, 134, 193, 0, 26, 139, 85], "identifier"=402391172, "type"=8, "extended?"=TRUE, "echo?"=FALSE}, "Read Session in"=w320, "Write Session in"=w321) -> ("TxRx Data"=w316:string[][])  [unwired: 1 in, 4 out]
        n129 = And(x=w338, y=w311) -> (x .and. y?=w336:bool)
        n130 = Build Array (concatenate)(w324, w317, w316) -> (w323:string[][])
        n131 = case shown="False" w311 {
          tunnel: w334 -> [w342 w344]
          tunnel: [w343 w344] -> w333
          tunnel: w328 -> [w341 _]
          frame False {
            n132 = Concatenate Strings(w342, w341) -> (w343:string)
          }
          frame True {
          }
        }
        n133 = Not(x=w311) -> (.not. x?=w312:bool)
        n134 = Bundle By Name(cluster=w337, "TxRx Data"=w323, "Response Good?"=w336, "Error String"=w333) -> (w335:T3)
        n135 = call "Insert Multiple Events.vi"("Insert all? (T)"=w312, "Events to Insert"=string[] ["Exit"], "Event queue in"=w326) -> ("Event queue out"=w327:string[])  [unwired: 4 in]
      }
      frame "Get Login Seed and Key" {
        n136 = Unbundle By Name(w365) -> ("Response Good?"=w366:bool, "TxRx Data"=w352:string[][], "Error String"=w362:string, "DSC Write Session in"=w348:refnum<k21>, "Read Session in"=w347:refnum<k21>, "Glass?"=w350:bool)
        n137 = Select(t=" - Glass" ("Error Description"), s=w350, f=" - Rollo" ("Error Description")) -> (s? t:f=w360:string)
        n138 = Concatenate Strings(w360, " - Get Login Seed and Key" ("Error Description")) -> (w356:string)
        n139 = call "EOL CAN_Get Seed and Key.vi"("Read Session in"=w347, "Write Session in"=w348) -> ("Response Good?"=w345:bool, "TxRx Data"=w346:string[][])  [unwired: 7 in, 1 out]
        n140 = And(x=w366, y=w345) -> (x .and. y?=w364:bool)
        n141 = Build Array (concatenate)(w352, w346) -> (w351:string[][])
        n142 = Not(x=w345) -> (.not. x?=w349:bool)
        n143 = case shown="False" w345 {
          tunnel: w362 -> [w368 w370]
          tunnel: [w369 w370] -> w361
          tunnel: w356 -> [w367 _]
          frame False {
            n144 = Concatenate Strings(w368, w367) -> (w369:string)
          }
          frame True {
          }
        }
        n145 = Bundle By Name(cluster=w365, "TxRx Data"=w351, "Response Good?"=w364, "Error String"=w361) -> (w363:T3)
        n146 = call "Insert Multiple Events.vi"("Insert all? (T)"=w349, "Events to Insert"=string[] ["Exit"], "Event queue in"=w354) -> ("Event queue out"=w355:string[])  [unwired: 4 in]
      }
      frame "Get Bootloader Seed and Key" {
        n147 = Unbundle By Name(w392) -> ("Response Good?"=w393:bool, "TxRx Data"=w379:string[][], "Error String"=w389:string, "DSC Write Session in"=w374:refnum<k21>, "Read Session in"=w373:refnum<k21>, "SA2 Operator"=w375:T1[], "Glass?"=w377:bool)
        n148 = Select(t=" - Glass" ("Error Description"), s=w377, f=" - Rollo" ("Error Description")) -> (s? t:f=w387:string)
        n149 = Concatenate Strings(w387, " - Get Bootloader Seed and Key" ("Error Description")) -> (w383:string)
        n150 = call "EOL CAN_Get Bootloader Key.vi"("SA2 Operator"=w375, "Read Session in"=w373, "Write Session in"=w374) -> ("Response Good?"=w371:bool, "TxRx Data"=w372:string[][])  [unwired: 6 in, 1 out]
        n151 = And(x=w393, y=w371) -> (x .and. y?=w391:bool)
        n152 = Build Array (concatenate)(w379, w372) -> (w378:string[][])
        n153 = Not(x=w371) -> (.not. x?=w376:bool)
        n154 = case shown="False" w371 {
          tunnel: w389 -> [w395 w397]
          tunnel: [w396 w397] -> w388
          tunnel: w383 -> [w394 _]
          frame False {
            n155 = Concatenate Strings(w395, w394) -> (w396:string)
          }
          frame True {
          }
        }
        n156 = Bundle By Name(cluster=w392, "TxRx Data"=w378, "Response Good?"=w391, "Error String"=w388) -> (w390:T3)
        n157 = call "Insert Multiple Events.vi"("Insert all? (T)"=w376, "Events to Insert"=string[] ["Exit"], "Event queue in"=w381) -> ("Event queue out"=w382:string[])  [unwired: 4 in]
      }
      frame "Enable Production Mode" {
        n158 = Unbundle By Name(w418) -> ("Response Good?"=w419:bool, "TxRx Data"=w405:string[][], "Error String"=w415:string, "DSC Write Session in"=w401:refnum<k21>, "Read Session in"=w400:refnum<k21>, "Glass?"=w403:bool)
        n159 = Select(t=" - Glass" ("Error Description"), s=w403, f=" - Rollo" ("Error Description")) -> (s? t:f=w413:string)
        n160 = Concatenate Strings(w413, " - Enable Production Mode" ("Error Description")) -> (w409:string)
        n161 = call "EOL CAN_Enable_Production_Mode.vi"("Read Session in"=w400, "Write Session in"=w401) -> ("debug log"=w399:string[][], "Response Good?"=w398:bool)  [unwired: 7 in, 1 out]
        n162 = And(x=w419, y=w398) -> (x .and. y?=w417:bool)
        n163 = Build Array (concatenate)(w405, w399) -> (w404:string[][])
        n164 = Not(x=w398) -> (.not. x?=w402:bool)
        n165 = case shown="False" w398 {
          tunnel: w415 -> [w421 w423]
          tunnel: [w422 w423] -> w414
          tunnel: w409 -> [w420 _]
          frame False {
            n166 = Concatenate Strings(w421, w420) -> (w422:string)
          }
          frame True {
          }
        }
        n167 = Bundle By Name(cluster=w418, "TxRx Data"=w404, "Response Good?"=w417, "Error String"=w414) -> (w416:T3)
        n168 = call "Insert Multiple Events.vi"("Insert all? (T)"=w402, "Events to Insert"=string[] ["Exit"], "Event queue in"=w407) -> ("Event queue out"=w408:string[])  [unwired: 4 in]
      }
      frame "Disable Production Mode" {
        n169 = Unbundle By Name(w444) -> ("Response Good?"=w445:bool, "TxRx Data"=w431:string[][], "Error String"=w441:string, "DSC Write Session in"=w427:refnum<k21>, "Read Session in"=w426:refnum<k21>, "Glass?"=w429:bool)
        n170 = Select(t=" - Glass" ("Error Description"), s=w429, f=" - Rollo" ("Error Description")) -> (s? t:f=w439:string)
        n171 = Concatenate Strings(w439, " - Disable Production Mode" ("Error Description")) -> (w435:string)
        n172 = call "EOL CAN_Disable_Production_Mode.vi"("Read Session in"=w426, "Write Session in"=w427) -> ("debug log"=w425:string[][], "Response Good?"=w424:bool)  [unwired: 7 in, 1 out]
        n173 = And(x=w445, y=w424) -> (x .and. y?=w443:bool)
        n174 = Build Array (concatenate)(w431, w425) -> (w430:string[][])
        n175 = Not(x=w424) -> (.not. x?=w428:bool)
        n176 = case shown="False" w424 {
          tunnel: w441 -> [w447 w449]
          tunnel: [w448 w449] -> w440
          tunnel: w435 -> [w446 _]
          frame False {
            n177 = Concatenate Strings(w447, w446) -> (w448:string)
          }
          frame True {
          }
        }
        n178 = Bundle By Name(cluster=w444, "TxRx Data"=w430, "Response Good?"=w443, "Error String"=w440) -> (w442:T3)
        n179 = call "Insert Multiple Events.vi"("Insert all? (T)"=w428, "Events to Insert"=string[] ["Exit"], "Event queue in"=w433) -> ("Event queue out"=w434:string[])  [unwired: 4 in]
      }
      frame "Set Programming Date" {
        n180 = Unbundle By Name(w481) -> ("Response Good?"=w482:bool, "TxRx Data"=w468:string[][], "Error String"=w478:string, "DSC Write Session in"=w464:refnum<k21>, "Read Session in"=w463:refnum<k21>, "Glass?"=w466:bool)
        n181 = Format Date/Time String(time format string (%c)="%y,%m,%d") -> (date/time string=w451:string)  [unwired: 2 in]
        n182 = Spreadsheet String To Array(delimiter (Tab)=",", format string="%x", spreadsheet string=w451, array type (2D Dbl)=u8[] []) -> (array=w450:u8[])
        n183 = Select(t=" - Glass" ("Error Description"), s=w466, f=" - Rollo" ("Error Description")) -> (s? t:f=w476:string)
        n184 = Replace Array Subset(array=u8[] [6, 46, 241, 153, 85, 85, 85, 85] ("payload"), new element=w450, index=4) -> (w457:u8[])
        n185 = Concatenate Strings(w476, " - Set Program Date" ("Error Description")) -> (w472:string)
        n186 = Bundle By Name(cluster=T5 {"timestamp"=timestamp(0 s since 1904-01-01), "payload"=[6, 46, 241, 153, 85, 85, 85, 85], "identifier"=402391172, "type"=8, "extended?"=TRUE, "echo?"=FALSE} ("Tx CAN frame"), "payload"=w457) -> (w459:T5)
        n187 = call "EOL CAN_Send_Single_Message.vi"("Tx CAN frame"=w459, "Read Session in"=w463, "Write Session in"=w464) -> ("Response Good?"=w461:bool, "TxRx Data"=w462:string[][])  [unwired: 4 in, 3 out]
        n188 = And(x=w482, y=w461) -> (x .and. y?=w480:bool)
        n189 = Build Array (concatenate)(w468, w462) -> (w467:string[][])
        n190 = Not(x=w461) -> (.not. x?=w465:bool)
        n191 = case shown="False" w461 {
          tunnel: w478 -> [w484 w486]
          tunnel: [w485 w486] -> w477
          tunnel: w472 -> [w483 _]
          frame False {
            n192 = Concatenate Strings(w484, w483) -> (w485:string)
          }
          frame True {
          }
        }
        n193 = Bundle By Name(cluster=w481, "TxRx Data"=w467, "Response Good?"=w480, "Error String"=w477) -> (w479:T3)
        n194 = call "Insert Multiple Events.vi"("Insert all? (T)"=w465, "Events to Insert"=string[] ["Exit"], "Event queue in"=w470) -> ("Event queue out"=w471:string[])  [unwired: 4 in]
      }
      frame "Set Start Routine 2" {
        n195 = Unbundle By Name(w511) -> ("Response Good?"=w512:bool, "TxRx Data"=w498:string[][], "Error String"=w508:string, "DSC Write Session in"=w494:refnum<k21>, "Read Session in"=w493:refnum<k21>, "Glass?"=w496:bool)
        n196 = flat-sequence {
          tunnel: [errorcluster {"status"=FALSE, "code"=0, "source"=""} ("Error in")] -> w487
          frame #0 {
            n197 = Wait (ms)(milliseconds to wait=u32 10) -> ()  [unwired: 1 out]
          }
        }
        n198 = Select(t=" - Glass" ("Error Description"), s=w496, f=" - Rollo" ("Error Description")) -> (s? t:f=w506:string)
        n199 = Concatenate Strings(w506, " - Set Program Date" ("Error Description")) -> (w502:string)
        n200 = call "EOL CAN_Send_Single_Message.vi"("Retries"=10, "Msg Wait Time"=u32 400, "Error in"=w487, "Tx CAN frame"=T5 {"timestamp"=timestamp(0 s since 1904-01-01), "payload"=[7, 49, 1, 255, 0, 2, 113, 0], "identifier"=402391172, "type"=8, "extended?"=TRUE, "echo?"=FALSE}, "Read Session in"=w493, "Write Session in"=w494) -> ("Response Good?"=w491:bool, "TxRx Data"=w492:string[][])  [unwired: 1 in, 3 out]
        n201 = And(x=w512, y=w491) -> (x .and. y?=w510:bool)
        n202 = Build Array (concatenate)(w498, w492) -> (w497:string[][])
        n203 = Not(x=w491) -> (.not. x?=w495:bool)
        n204 = case shown="False" w491 {
          tunnel: w508 -> [w516 w518]
          tunnel: [w517 w518] -> w507
          tunnel: w502 -> [w515 _]
          frame False {
            n205 = Concatenate Strings(w516, w515) -> (w517:string)
          }
          frame True {
          }
        }
        n206 = Bundle By Name(cluster=w511, "TxRx Data"=w497, "Response Good?"=w510, "Error String"=w507) -> (w509:T3)
        n207 = call "Insert Multiple Events.vi"("Insert all? (T)"=w495, "Events to Insert"=string[] ["Exit"], "Event queue in"=w500) -> ("Event queue out"=w501:string[])  [unwired: 4 in]
      }
      frame "Set Blah 2" {
        n208 = Unbundle By Name(w542) -> ("Response Good?"=w543:bool, "TxRx Data"=w529:string[][], "Error String"=w539:string, "DSC Write Session in"=w525:refnum<k21>, "Read Session in"=w524:refnum<k21>, "Glass?"=w527:bool)
        n209 = Select(t=" - Glass" ("Error Description"), s=w527, f=" - Rollo" ("Error Description")) -> (s? t:f=w537:string)
        n210 = Concatenate Strings(w537, " - Set Program Date" ("Error Description")) -> (w533:string)
        n211 = call "EOL CAN_Send_Single_Message.vi"("Retries"=10, "Msg Wait Time"=u32 100, "Tx CAN frame"=T5 {"timestamp"=timestamp(0 s since 1904-01-01), "payload"=[7, 46, 241, 161, 48, 48, 48, 48], "identifier"=402391172, "type"=8, "extended?"=TRUE, "echo?"=FALSE}, "Read Session in"=w524, "Write Session in"=w525) -> ("Response Good?"=w519:bool, "TxRx Data"=w523:string[][])  [unwired: 2 in, 3 out]
        n212 = And(x=w543, y=w519) -> (x .and. y?=w541:bool)
        n213 = Build Array (concatenate)(w529, w523) -> (w528:string[][])
        n214 = Not(x=w519) -> (.not. x?=w526:bool)
        n215 = case shown="False" w519 {
          tunnel: w539 -> [w545 w547]
          tunnel: [w546 w547] -> w538
          tunnel: w533 -> [w544 _]
          frame False {
            n216 = Concatenate Strings(w545, w544) -> (w546:string)
          }
          frame True {
          }
        }
        n217 = Bundle By Name(cluster=w542, "TxRx Data"=w528, "Response Good?"=w541, "Error String"=w538) -> (w540:T3)
        n218 = call "Insert Multiple Events.vi"("Insert all? (T)"=w526, "Events to Insert"=string[] ["Exit"], "Event queue in"=w531) -> ("Event queue out"=w532:string[])  [unwired: 4 in]
      }
      frame "Set Blah 3" {
        w548 = TRUE ("y")
        n219 = Unbundle By Name(w571) -> ("Response Good?"=w572:bool, "TxRx Data"=w558:string[][], "Error String"=w568:string, "DSC Write Session in"=w554:refnum<k21>, "Read Session in"=w553:refnum<k21>, "Glass?"=w556:bool)
        n220 = Select(t=" - Glass" ("Error Description"), s=w556, f=" - Rollo" ("Error Description")) -> (s? t:f=w566:string)
        n221 = Concatenate Strings(w566, " - Set Program Date" ("Error Description")) -> (w562:string)
        n222 = call "EOL CAN_Send_Single_Message.vi"("Retries"=10, "Msg Wait Time"=u32 100, "Tx CAN frame"=T5 {"timestamp"=timestamp(0 s since 1904-01-01), "payload"=[3, 40, 1, 1, 85, 85, 85, 85], "identifier"=402391172, "type"=8, "extended?"=TRUE, "echo?"=FALSE}, "Read Session in"=w553, "Write Session in"=w554) -> ("TxRx Data"=w552:string[][])  [unwired: 2 in, 4 out]
        n223 = And(x=w572, y=w548) -> (x .and. y?=w570:bool)
        n224 = Build Array (concatenate)(w558, w552) -> (w557:string[][])
        n225 = Not(x=w548) -> (.not. x?=w555:bool)
        n226 = case shown="False" w548 {
          tunnel: w568 -> [w574 w576]
          tunnel: [w575 w576] -> w567
          tunnel: w562 -> [w573 _]
          frame False {
            n227 = Concatenate Strings(w574, w573) -> (w575:string)
          }
          frame True {
          }
        }
        n228 = Bundle By Name(cluster=w571, "TxRx Data"=w557, "Response Good?"=w570, "Error String"=w567) -> (w569:T3)
        n229 = call "Insert Multiple Events.vi"("Insert all? (T)"=w555, "Events to Insert"=string[] ["Exit"], "Event queue in"=w560) -> ("Event queue out"=w561:string[])  [unwired: 4 in]
      }
      frame "Set Start Routine 1" {
        w577 = TRUE
        n230 = Unbundle By Name(w598) -> ("Response Good?"=w599:bool, "TxRx Data"=w585:string[][], "Error String"=w595:string, "DSC Write Session in"=w581:refnum<k21>, "Read Session in"=w580:refnum<k21>, "Glass?"=w583:bool)
        n231 = Select(t=" - Glass" ("Error Description"), s=w583, f=" - Rollo" ("Error Description")) -> (s? t:f=w593:string)
        n232 = Concatenate Strings(w593, " - Set Program Date" ("Error Description")) -> (w589:string)
        n233 = call "EOL CAN_Send_Single_Message.vi"("Tx CAN frame"=T5 {"timestamp"=timestamp(0 s since 1904-01-01), "payload"=[4, 49, 1, 2, 3, 85, 85, 85], "identifier"=402391172, "type"=8, "extended?"=TRUE, "echo?"=FALSE}, "Read Session in"=w580, "Write Session in"=w581) -> ("TxRx Data"=w579:string[][])  [unwired: 4 in, 4 out]
        n234 = And(x=w599, y=w577) -> (x .and. y?=w597:bool)
        n235 = Build Array (concatenate)(w585, w579) -> (w584:string[][])
        n236 = Not(x=w577) -> (.not. x?=w582:bool)
        n237 = case shown="False" w577 {
          tunnel: w595 -> [w601 w603]
          tunnel: [w602 w603] -> w594
          tunnel: w589 -> [w600 _]
          frame False {
            n238 = Concatenate Strings(w601, w600) -> (w602:string)
          }
          frame True {
          }
        }
        n239 = Bundle By Name(cluster=w598, "TxRx Data"=w584, "Response Good?"=w597, "Error String"=w594) -> (w596:T3)
        n240 = call "Insert Multiple Events.vi"("Insert all? (T)"=w582, "Events to Insert"=string[] ["Exit"], "Event queue in"=w587) -> ("Event queue out"=w588:string[])  [unwired: 4 in]
      }
      frame "Activate Development Frames" {
        n241 = Unbundle By Name(w625) -> ("Response Good?"=w626:bool, "TxRx Data"=w612:string[][], "Error String"=w622:string, "DSC Write Session in"=w608:refnum<k21>, "Read Session in"=w607:refnum<k21>, "Glass?"=w610:bool)
        n242 = Select(t=" - Glass" ("Error Description"), s=w610, f=" - Rollo" ("Error Description")) -> (s? t:f=w620:string)
        n243 = Concatenate Strings(w620, " - Activate Dev Frames" ("Error Description")) -> (w616:string)
        n244 = call "EOL CAN_Send_Single_Message.vi"("Tx CAN frame"=T5 {"timestamp"=timestamp(0 s since 1904-01-01), "payload"=[4, 46, 9, 2, 128, 85, 85, 85], "identifier"=402391172, "type"=8, "extended?"=TRUE, "echo?"=FALSE}, "Read Session in"=w607, "Write Session in"=w608) -> ("Response Good?"=w605:bool, "TxRx Data"=w606:string[][])  [unwired: 4 in, 3 out]
        n245 = And(x=w626, y=w605) -> (x .and. y?=w624:bool)
        n246 = Build Array (concatenate)(w612, w606) -> (w611:string[][])
        n247 = Not(x=w605) -> (.not. x?=w609:bool)
        n248 = case shown="False" w605 {
          tunnel: w622 -> [w628 w630]
          tunnel: [w629 w630] -> w621
          tunnel: w616 -> [w627 _]
          frame False {
            n249 = Concatenate Strings(w628, w627) -> (w629:string)
          }
          frame True {
          }
        }
        n250 = Bundle By Name(cluster=w625, "TxRx Data"=w611, "Response Good?"=w624, "Error String"=w621) -> (w623:T3)
        n251 = call "Insert Multiple Events.vi"("Insert all? (T)"=w609, "Events to Insert"=string[] ["Exit"], "Event queue in"=w614) -> ("Event queue out"=w615:string[])  [unwired: 4 in]
      }
      frame "Set Key Off On Reset" {
        n252 = Unbundle By Name(w652) -> ("Response Good?"=w653:bool, "TxRx Data"=w639:string[][], "Error String"=w649:string, "DSC Write Session in"=w635:refnum<k21>, "Read Session in"=w634:refnum<k21>, "Glass?"=w637:bool)
        n253 = Select(t=" - Glass" ("Error Description"), s=w637, f=" - Rollo" ("Error Description")) -> (s? t:f=w647:string)
        n254 = Concatenate Strings(w647, " - Key Off On Reset" ("Error Description")) -> (w643:string)
        n255 = call "EOL CAN_Send_Single_Message.vi"("Tx CAN frame"=T5 {"timestamp"=timestamp(0 s since 1904-01-01), "payload"=[2, 17, 2, 85, 85, 85, 85, 85], "identifier"=402391172, "type"=8, "extended?"=TRUE, "echo?"=FALSE}, "Read Session in"=w634, "Write Session in"=w635) -> ("Response Good?"=w632:bool, "TxRx Data"=w633:string[][])  [unwired: 4 in, 3 out]
        n256 = And(x=w653, y=w632) -> (x .and. y?=w651:bool)
        n257 = Build Array (concatenate)(w639, w633) -> (w638:string[][])
        n258 = Not(x=w632) -> (.not. x?=w636:bool)
        n259 = case shown="False" w632 {
          tunnel: w649 -> [w655 w657]
          tunnel: [w656 w657] -> w648
          tunnel: w643 -> [w654 _]
          frame False {
            n260 = Concatenate Strings(w655, w654) -> (w656:string)
          }
          frame True {
          }
        }
        n261 = Bundle By Name(cluster=w652, "TxRx Data"=w638, "Response Good?"=w651, "Error String"=w648) -> (w650:T3)
        n262 = call "Insert Multiple Events.vi"("Insert all? (T)"=w636, "Events to Insert"=string[] ["Exit"], "Event queue in"=w641) -> ("Event queue out"=w642:string[])  [unwired: 4 in]
      }
      frame "Clear DTC" {
        n263 = Unbundle By Name(w678) -> ("Response Good?"=w679:bool, "TxRx Data"=w665:string[][], "Error String"=w675:string, "DSC Write Session in"=w661:refnum<k21>, "Read Session in"=w660:refnum<k21>, "Glass?"=w663:bool)
        n264 = Select(t=" - Glass" ("Error Description"), s=w663, f=" - Rollo" ("Error Description")) -> (s? t:f=w673:string)
        n265 = Concatenate Strings(w673, " - Clear DTC" ("Error Description")) -> (w669:string)
        n266 = call "EOL CAN_Clear_DTC's.vi"("Read Session in"=w660, "Write Session in"=w661) -> ("TxRx Data"=w659:string[][], "Response Good?"=w658:bool)  [unwired: 7 in, 1 out]
        n267 = And(x=w679, y=w658) -> (x .and. y?=w677:bool)
        n268 = Build Array (concatenate)(w665, w659) -> (w664:string[][])
        n269 = Not(x=w658) -> (.not. x?=w662:bool)
        n270 = case shown="False" w658 {
          tunnel: w675 -> [w681 w683]
          tunnel: [w682 w683] -> w674
          tunnel: w669 -> [w680 _]
          frame False {
            n271 = Concatenate Strings(w681, w680) -> (w682:string)
          }
          frame True {
          }
        }
        n272 = Bundle By Name(cluster=w678, "TxRx Data"=w664, "Response Good?"=w677, "Error String"=w674) -> (w676:T3)
        n273 = call "Insert Multiple Events.vi"("Insert all? (T)"=w662, "Events to Insert"=string[] ["Exit"], "Event queue in"=w667) -> ("Event queue out"=w668:string[])  [unwired: 4 in]
      }
      frame "Exit" {
        n274 = Unbundle By Name(w687) -> ("Response Good?"=→"Response Good?":bool, "Error String"=→"Error String Out":string, "TxRx Data"=→"TxRx Data":string[][])
      }
    }
  }
